vi "DDS Comms.vi"(7 "Config Folder":path, 8 "error in":errorcluster, 9 "DVR":T1, 10 "DDS Reader":refnum<class "DDS Reader.lvclass">, 11 "DDS Writer":refnum<class "DDS Writer.lvclass">) -> (0 "error out":errorcluster)   [LabVIEW 2018]
uses:
  Controls/Data Type DVRs.ctl
  <vilib>/ORNL/CSEISMIC DDS/DDS Writer/DDS Writer.lvclass
  C:/Program Files (x86)/National Instruments/LabVIEW 2018/vi.lib/ORNL/CSEISMIC DDS/CSEISMIC DDS Base/CSEISMIC DDS.lvclass
  <vilib>/ORNL/CSEISMIC DDS/DDS Reader/DDS Reader.lvclass
  <vilib>/ORNL/CSEISMIC DDS/CSEISMIC DDS Base/Data Types/IED_Status.ctl
  <vilib>/ORNL/CSEISMIC DDS/CSEISMIC DDS Base/Data Types/Controls/DeviceID.ctl
  <vilib>/ORNL/CSEISMIC DDS/CSEISMIC DDS Base/Data Types/Controls/Timestamp.ctl
  <vilib>/ORNL/CSEISMIC DDS/CSEISMIC DDS Base/Data Types/DER_Status.ctl
  <vilib>/ORNL/CSEISMIC DDS/CSEISMIC DDS Base/Data Types/Controls/DroopCurve.ctl
  <vilib>/ORNL/CSEISMIC DDS/CSEISMIC DDS Base/Data Types/DER_Info.ctl
  <vilib>/ORNL/CSEISMIC DDS/CSEISMIC DDS Base/Data Types/DER_Measurement.ctl
  <vilib>/ORNL/CSEISMIC DDS/CSEISMIC DDS Base/Data Types/ES_Info.ctl
  <vilib>/ORNL/CSEISMIC DDS/CSEISMIC DDS Base/Data Types/Controls/EfficiencyCurve.ctl
  <vilib>/ORNL/CSEISMIC DDS/CSEISMIC DDS Base/Data Types/ES_Measurement.ctl
  <vilib>/ORNL/CSEISMIC DDS/CSEISMIC DDS Base/Data Types/Generator_Info.ctl
  <vilib>/ORNL/CSEISMIC DDS/CSEISMIC DDS Base/Data Types/DER_setGenerationMode.ctl
  <vilib>/ORNL/CSEISMIC DDS/CSEISMIC DDS Base/Data Types/Controls/Generation Mode.ctl
  <vilib>/ORNL/CSEISMIC DDS/CSEISMIC DDS Base/Data Types/SmartRelay_Info.ctl
  <vilib>/ORNL/CSEISMIC DDS/CSEISMIC DDS Base/Data Types/SmartRelay_Measurement.ctl
  <vilib>/ORNL/CSEISMIC DDS/CSEISMIC DDS Base/CSEISMIC DDS.lvclass/CSEISMIC DDS.ctl
  74af6b33-939e-4f48-b39b-7a03e9a3d2c4.vi
  925c311d-217e-4777-a47a-50ede28ddcd3.vi
  1b66878a-8a8f-45b3-9ec7-57a0231460af.vi
  15938f2e-ac62-4bfc-b10c-904afcaf9918.vi
  fedd38d1-ecdd-43ef-a46f-a7af2de55406.vi
  6013e8e3-4859-43dd-bd06-f29373650741.vi
  0c0dbf40-5b73-4af0-b989-68fcfa5814cd.vi
  ee962d0e-06f6-400d-86d6-c1f49f22facc.vi
  943a1034-7167-4452-8124-675b30d37505.vi
  90619f50-e501-428c-b219-0f596dcd4826.vi
  a52a024a-1226-4015-a4cd-490690dd4f10.vi
  0e523b0e-f060-4810-9406-aaa83c92bbf0.vi
  bea21f4c-5d2d-47b9-9a7d-942307ba0c0f.vi
  88d5637e-ab37-41e7-8b27-781a427d1398.vi
  068224fe-cff3-42fe-a570-2705411094f8.vi
  62cf694c-65b3-493c-badd-292e3eb2e763.vi
  20c1c1fb-87c8-4a1b-abc1-d694dbcccceb.vi
  458aed31-5bcb-498f-bb6f-82a7e59887fc.vi
  6bb0f422-3d80-46dd-aaf7-aed45feee7e6.vi
  d6538dc3-a141-461a-88df-898e5ba76e67.vi
  <vilib>/ORNL/CSEISMIC DDS/CSEISMIC DDS Base/Accessors/Read DDS Reference.vi
  <vilib>/Utility/config.llb/Read Key (String).vi
  Global Variables/Stop (Global).vi
  <vilib>/ORNL/CSEISMIC DDS/CSEISMIC DDS Base/Error Handler.vi
  <vilib>/ORNL/CSEISMIC DDS/CSEISMIC DDS Base/CSEISMIC DDS.lvclass
  <vilib>/Utility/config.llb/NI_LVConfig.lvlib
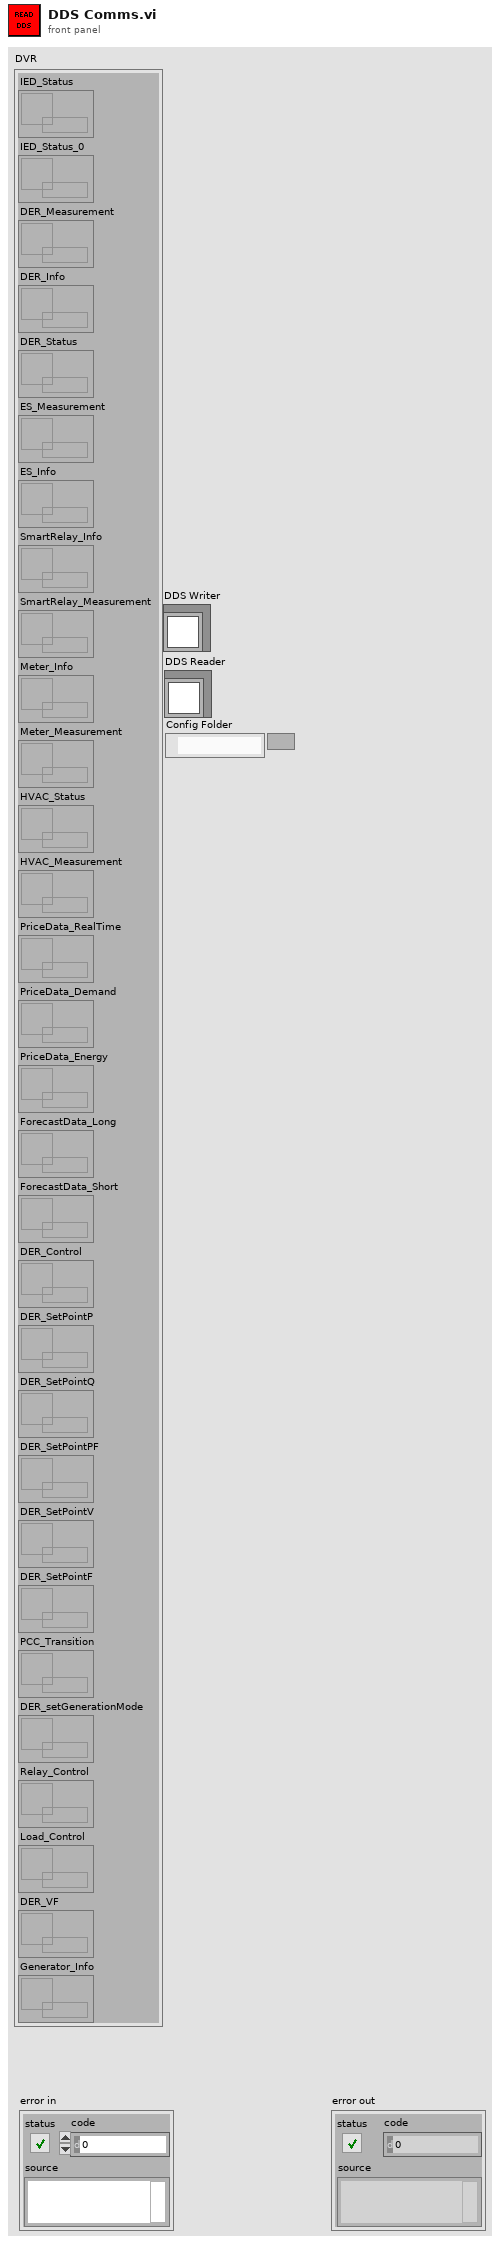
[diagram p1: front panel]
types:
  T1 = typedef "Data Type DVRs.ctl" = cluster{"IED_Status":refnum<data-value>, "IED_Status_0":refnum<data-value>, "DER_Measurement":refnum<data-value>, "DER_Info":refnum<data-value>, "DER_Status":refnum<data-value>, "ES_Measurement":refnum<data-value>, "ES_Info":refnum<data-value>, "SmartRelay_Info":refnum<data-value>, "SmartRelay_Measurement":refnum<data-value>, "Meter_Info":refnum<data-value>, "Meter_Measurement":refnum<data-value>, "HVAC_Status":refnum<data-value>, "HVAC_Measurement":refnum<data-value>, "PriceData_RealTime":refnum<data-value>, "PriceData_Demand":refnum<data-value>, "PriceData_Energy":refnum<data-value>, "ForecastData_Long":refnum<data-value>, "ForecastData_Short":refnum<data-value>, "DER_Control":refnum<data-value>, "DER_SetPointP":refnum<data-value>, "DER_SetPointQ":refnum<data-value>, "DER_SetPointPF":refnum<data-value>, "DER_SetPointV":refnum<data-value>, "DER_SetPointF":refnum<data-value>, "PCC_Transition":refnum<data-value>, "DER_setGenerationMode":refnum<data-value>, "Relay_Control":refnum<data-value>, "Load_Control":refnum<data-value>, "DER_VF":refnum<data-value>, "Generator_Info":refnum<data-value>}
  T2 = typedef "NI_LVConfig.lvlib/Config Data RefNum.ctl" = refnum<k1>
  T3 = typedef "CSEISMIC DDS.lvlib/CSEISMIC DDS.lvclass/SmartRelay_Measurement.ctl" = cluster{"DeviceID":T4, "PrimaryVoltage":dbl[], "SecondaryVoltage":dbl[], "Current":dbl[], "RealPower":dbl[], "ReactivePower":dbl[], "LineConfig":u8[], "Frequency":dbl}
  T4 = typedef "CSEISMIC DDS.lvlib/CSEISMIC DDS.lvclass/DeviceID.ctl" = string
  T5 = typedef "CSEISMIC DDS.lvlib/CSEISMIC DDS.lvclass/SmartRelay_Info.ctl" = cluster{"DeviceID":T4, "LineConfig":u8[], "NominalVoltage(V)":dbl}
  T6 = typedef "CSEISMIC DDS.lvlib/CSEISMIC DDS.lvclass/DER_setGenerationMode.ctl" = cluster{"DeviceID":T4, "Mode":T7}
  T7 = typedef "CSEISMIC DDS.lvlib/CSEISMIC DDS.lvclass/Generation Mode.ctl" = enum32{"Invalid", "PQ", "Droop", "PV", "PF", "VF"}
  T8 = typedef "CSEISMIC DDS.lvlib/CSEISMIC DDS.lvclass/Generator_Info.ctl" = cluster{"DeviceID":T4, "Voltage (V)":dbl, "MinimumPower (kVA)":dbl, "EnergyRating (kWh)":dbl, "RampRate (kW/s)":dbl, "MaxPowerFactorLeading":dbl, "MaxPowerFactorLagging":dbl, "EfficiencyCurve":T9, "StartCost":dbl, "FuelCost":dbl, "StartTime (s)":dbl}
  T9 = typedef "CSEISMIC DDS.lvlib/CSEISMIC DDS.lvclass/EfficiencyCurve.ctl" = cluster{"Power (kW)":dbl[], "Efficiency (%)":dbl[]}
  T10 = typedef "CSEISMIC DDS.lvlib/CSEISMIC DDS.lvclass/ES_Measurement.ctl" = cluster{"DeviceID":T4, "SOC (%)":dbl}
  T11 = typedef "CSEISMIC DDS.lvlib/CSEISMIC DDS.lvclass/ES_Info.ctl" = cluster{"DeviceID":T4, "EnergyRating (kWh)":dbl, "RampRate (kW/s)":dbl, "MaxPowerFactorLeading":dbl, "MaxPowerFactorLagging":dbl, "ChargingEfficiencyCurve":T9, "DischargingEfficiencyCurve":T9, "MinSOC (%)":dbl, "MaxSOC (%)":dbl}
  T12 = typedef "CSEISMIC DDS.lvlib/CSEISMIC DDS.lvclass/DER_Measurement.ctl" = cluster{"DeviceID":T4, "Voltage":dbl[], "Current":dbl[], "RealPower":dbl[], "ReactivePower":dbl[], "LineConfig":u8[], "Frequency":dbl}
  T13 = typedef "CSEISMIC DDS.lvlib/CSEISMIC DDS.lvclass/DER_Info.ctl" = cluster{"DeviceID":T4, "LineConfig":u8[], "NominalVoltage(V)":dbl, "PowerRating(kVA)":dbl, "VFControl":bool, "PControl":bool, "QControl":bool, "PFControl":bool, "PVControl":bool, "Droop":bool, "DroopConfigurable":bool, "Unbalanced":bool}
  T14 = typedef "CSEISMIC DDS.lvlib/CSEISMIC DDS.lvclass/DER_Status.ctl" = cluster{"DeviceID":T4, "VFControl":bool, "PControl":bool, "QControl":bool, "PFControl":bool, "PVControl":bool, "Droop":bool, "Unbalanced":bool, "MicrogridVF":bool, "RealDroop(kW)":T15, "ReactiveDroop(kVar)":T15}
  T15 = typedef "CSEISMIC DDS.lvlib/CSEISMIC DDS.lvclass/DroopCurve.ctl" = cluster{"XMin":dbl, "XMax":dbl, "YMin":dbl, "YMax":dbl}
  T16 = typedef "CSEISMIC DDS.lvlib/CSEISMIC DDS.lvclass/IED_Status.ctl" = cluster{"DeviceID":T4, "Timestamp":T17, "MicrogridID":u8, "Active":bool, "Inactive":bool, "Error":i32, "Fault":bool, "ErrorString":string}
  T17 = typedef "CSEISMIC DDS.lvlib/CSEISMIC DDS.lvclass/Timestamp.ctl" = cluster{"Seconds":u64, "Remainder":u64}
  T18 = typedef "CSEISMIC DDS.lvlib/CSEISMIC DDS.lvclass/DER_Control.ctl" = cluster{"DeviceID":T4, "Activate":bool, "Deactivate":bool}
  T19 = typedef "LVDDS_library.lvlib/DDS Sample Info.ctl" = cluster{"DDS_SampleStateKind":enum32{"DDS_INVALID_SAMPLE_STATE", "DDS_READ_SAMPLE_STATE", "DDS_NOT_READ_SAMPLE_STATE"}, "DDS_ViewStateKind":enum32{"DDS_INVALID_SAMPLE_STATE", "DDS_NEW_VIEW_STATE", "DDS_NOT_NEW_VIEW_STATE"}, "DDS_InstanceStateKind":enum32{"DDS_INVALID_STATE", "DDS_ALIVE_INSTANCE_STATE", "DDS_NOT_ALIVE_DISPOSED_INSTANCE_STATE", "", "DDS_NOT_ALIVE_NO_WRITERS_INSTANCE_STATE"}, "sec":i32, "nanosec":u32, "valid_data":bool}
  T20 = typedef "CSEISMIC DDS.lvlib/CSEISMIC DDS.lvclass/PCC_Transition.ctl" = cluster{"DeviceID":T4, "Island":bool, "Resynchronize":bool}
  T21 = typedef "CSEISMIC DDS.lvlib/CSEISMIC DDS.lvclass/DER_SetPointP.ctl" = cluster{"DeviceID":T4, "RealPower (kW)":dbl[]}
  T22 = typedef "CSEISMIC DDS.lvlib/CSEISMIC DDS.lvclass/DER_SetPointQ.ctl" = cluster{"DeviceID":T4, "ReactivePower (kVAR)":dbl[]}
  T23 = typedef "CSEISMIC DDS.lvlib/CSEISMIC DDS.lvclass/DER_SetPointF.ctl" = cluster{"DeviceID":T4, "Frequency (Hz)":dbl}
  T24 = typedef "CSEISMIC DDS.lvlib/CSEISMIC DDS.lvclass/DER_SetPointV.ctl" = cluster{"DeviceID":T4, "Voltage (V)":dbl}
  T25 = typedef "CSEISMIC DDS.lvlib/CSEISMIC DDS.lvclass/DER_VF.ctl" = cluster{"DeviceID":T4}
  T26 = typedef "CSEISMIC DDS.lvlib/CSEISMIC DDS.lvclass/Relay_Control.ctl" = cluster{"DeviceID":T4, "Activate":bool, "Deactivate":bool}
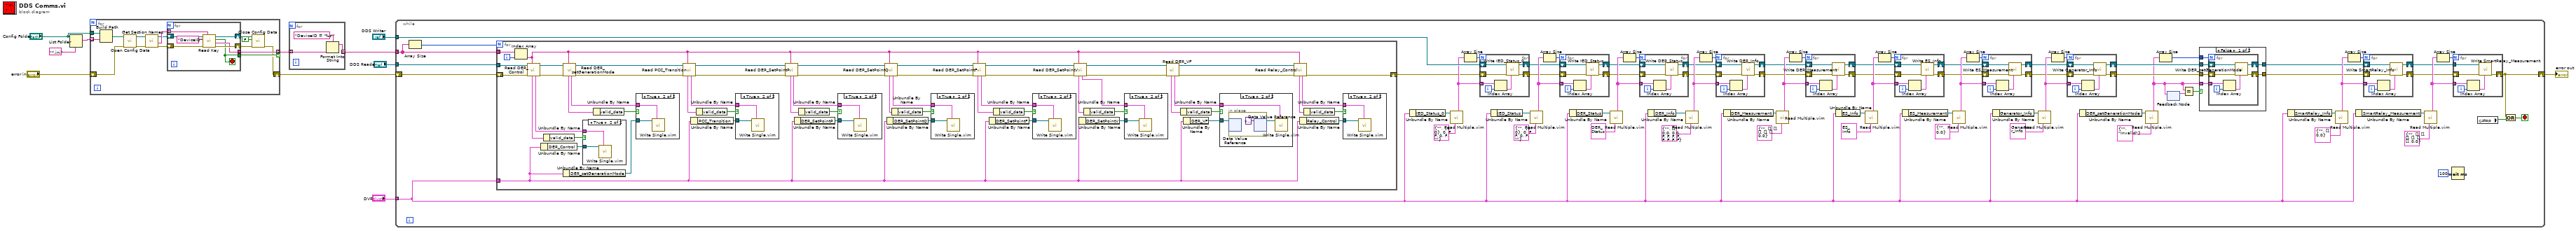
[diagram p0: block diagram]
diagram:
  n1 = List Folder(path="Config Folder", pattern="*.ini") -> (filenames=w5:string[])  [unwired: 2 in, 3 out]
  n2 = for {
    tunnel: w5 -> [w25] mode=indexing
    tunnel: "Config Folder" -> [w26]
    shift-right: [w13] -> w1
    shift-left: "error in" -> [w21]
    tunnel: [w17] -> w2 mode=indexing if=w14
    n3 = Build Path(base path=w26, name or relative path=w25) -> (appended path=w22:path)
    n4 = call <vilib>:"Open Config Data.vi"("error in (no error)"=w21, "configuration file path"=w22) -> ("error out"=w24:errorcluster, "refnum"=w23:T2)  [unwired: 7 in, 1 out]
    n5 = call <vilib>:"Get Section Names.vi"("error in (no error)"=w24, "refnum"=w23) -> ("error out"=w18:errorcluster, "section names"=w20:string[], "refnum out"=w19:T2)  [unwired: 7 in]
    n6 = for {
      tunnel: w20 -> [w34] mode=indexing
      shift-right: [w30] -> w16
      shift-left: w19 -> [w33]
      shift-right: [w31] -> w15
      shift-left: w18 -> [w32]
      tunnel: [w28] -> w17
      tunnel: [w27] -> w14
      stop <- w27 stop-if-true
      n7 = call-poly <vilib>:"Read Key.vi"("section"=w34, "error in (no error)"=w32, "key"="DeviceID", "refnum"=w33) -> ("error out"=w31:errorcluster, "value"=w28:string, "found?"=w27:bool, "refnum out"=w30:T2)  [unwired: 4 in]
    }
    n8 = call <vilib>:"Close Config Data.vi"("error in (no error)"=w15, "write file if changed (T)"=FALSE, "refnum"=w16) -> ("error out"=w13:errorcluster)  [unwired: 7 in, 1 out]
  }
  n9 = for {
    tunnel: w2 -> [w36] mode=indexing
    tunnel: [w35] -> w7 mode=indexing
    n10 = Format Into String(format string="DeviceID = '%s'" ("Query condition"), w36) -> (resulting string=w35:string)  [unwired: 2 in, 1 out]
  }
  n11 = while {
    tunnel: "DDS Reader" -> [w114]
    tunnel: "DDS Writer" -> [w112]
    tunnel: "DVR" -> [w93]
    shift-right: [w41] -> w10
    shift-left: w1 -> [w113]
    tunnel: w7 -> [w85]
    stop <- w87 stop-if-true
    n12 = Array Size(array=w85) -> (size(s)=w84:i32)
    n13 = for {
      N: w84 -> [_]
      tunnel: w114 -> [w171]
      tunnel: w93 -> [w116]
      shift-right: [w129] -> w70
      shift-left: w113 -> [w128]
      tunnel: w85 -> [w127]
      i -> [w126]
      n14 = Index Array(array=w127, index=w126) -> (element=w119:string)
      n15 = call <vilib>:"Read DER_Control.vi"("Query condition"=w119, "error in"=w128, "DDS Reader in"=w171) -> ("error out"=w173:errorcluster, "DDS Reader out"=w172:refnum<class "DDS Reader.lvclass">, "data"=w157:T18, "DDS Sample Info"=w159:T19)  [unwired: 5 in]
      n16 = Unbundle By Name(w116) -> ("DER_Control"=w160:refnum<data-value>)
      n17 = Unbundle By Name(w159) -> ("valid_data"=w158:bool)
      n18 = Unbundle By Name(w116) -> ("DER_setGenerationMode"=w155:refnum<data-value>)
      n19 = call <vilib>:"Read DER_setGenerationMode.vi"("Query condition"=w119, "error in"=w173, "DDS Reader in"=w172) -> ("error out"=w169:errorcluster, "DDS Reader out"=w170:refnum<class "DDS Reader.lvclass">, "data"=w154:T6, "DDS Sample Info"=w153:T19)  [unwired: 5 in]
      n20 = case shown="True" w158 {
        tunnel: w160 -> [_ w191]
        tunnel: w157 -> [_ w190]
        frame False {
        }
        frame True {
          n21 = call "Write Single.vim"("Data Element"=w190, "Data DVR"=w191) -> ()  [unwired: 9 in, 1 out]
        }
      }
      n22 = Unbundle By Name(w153) -> ("valid_data"=w156:bool)
      n23 = case shown="True" w156 {
        tunnel: w155 -> [_ w189]
        tunnel: w154 -> [_ w188]
        frame False {
        }
        frame True {
          n24 = call "Write Single.vim"("Data Element"=w188, "Data DVR"=w189) -> ()  [unwired: 9 in, 1 out]
        }
      }
      n25 = call <vilib>:"Read PCC_Transition.vi"("Query condition"=w119, "error in"=w169, "DDS Reader in"=w170) -> ("error out"=w168:errorcluster, "DDS Reader out"=w167:refnum<class "DDS Reader.lvclass">, "data"=w150:T20, "DDS Sample Info"=w149:T19)  [unwired: 5 in]
      n26 = Unbundle By Name(w116) -> ("PCC_Transition"=w151:refnum<data-value>)
      n27 = Unbundle By Name(w149) -> ("valid_data"=w152:bool)
      n28 = case shown="True" w152 {
        tunnel: w151 -> [_ w183]
        tunnel: w150 -> [_ w182]
        frame False {
        }
        frame True {
          n29 = call "Write Single.vim"("Data Element"=w182, "Data DVR"=w183) -> ()  [unwired: 9 in, 1 out]
        }
      }
      n30 = call <vilib>:"Read DER_SetPointP.vi"("Query condition"=w119, "error in"=w168, "DDS Reader in"=w167) -> ("error out"=w165:errorcluster, "DDS Reader out"=w166:refnum<class "DDS Reader.lvclass">, "data"=w146:T21, "DDS Sample Info"=w145:T19)  [unwired: 5 in]
      n31 = Unbundle By Name(w116) -> ("DER_SetPointP"=w148:refnum<data-value>)
      n32 = Unbundle By Name(w145) -> ("valid_data"=w147:bool)
      n33 = case shown="True" w147 {
        tunnel: w148 -> [_ w181]
        tunnel: w146 -> [_ w180]
        frame False {
        }
        frame True {
          n34 = call "Write Single.vim"("Data Element"=w180, "Data DVR"=w181) -> ()  [unwired: 9 in, 1 out]
        }
      }
      n35 = call <vilib>:"Read DER_SetPointQ.vi"("Query condition"=w119, "error in"=w165, "DDS Reader in"=w166) -> ("error out"=w163:errorcluster, "DDS Reader out"=w164:refnum<class "DDS Reader.lvclass">, "data"=w142:T22, "DDS Sample Info"=w141:T19)  [unwired: 5 in]
      n36 = Unbundle By Name(w116) -> ("DER_SetPointQ"=w143:refnum<data-value>)
      n37 = Unbundle By Name(w141) -> ("valid_data"=w144:bool)
      n38 = case shown="True" w144 {
        tunnel: w143 -> [_ w185]
        tunnel: w142 -> [_ w184]
        frame False {
        }
        frame True {
          n39 = call "Write Single.vim"("Data Element"=w184, "Data DVR"=w185) -> ()  [unwired: 9 in, 1 out]
        }
      }
      n40 = call <vilib>:"Read DER_SetPointF.vi"("Query condition"=w119, "error in"=w163, "DDS Reader in"=w164) -> ("error out"=w121:errorcluster, "DDS Reader out"=w123:refnum<class "DDS Reader.lvclass">, "data"=w115:T23, "DDS Sample Info"=w138:T19)  [unwired: 5 in]
      n41 = Unbundle By Name(w116) -> ("DER_SetPointF"=w140:refnum<data-value>)
      n42 = Unbundle By Name(w138) -> ("valid_data"=w139:bool)
      n43 = case shown="True" w139 {
        tunnel: w140 -> [_ w187]
        tunnel: w115 -> [_ w186]
        frame False {
        }
        frame True {
          n44 = call "Write Single.vim"("Data Element"=w186, "Data DVR"=w187) -> ()  [unwired: 9 in, 1 out]
        }
      }
      n45 = call <vilib>:"Read DER_SetPointV.vi"("Query condition"=w119, "error in"=w121, "DDS Reader in"=w123) -> ("error out"=w120:errorcluster, "DDS Reader out"=w122:refnum<class "DDS Reader.lvclass">, "data"=w117:T24, "DDS Sample Info"=w118:T19)  [unwired: 5 in]
      n46 = Unbundle By Name(w116) -> ("DER_SetPointV"=w124:refnum<data-value>)
      n47 = Unbundle By Name(w118) -> ("valid_data"=w125:bool)
      n48 = case shown="True" w125 {
        tunnel: w124 -> [_ w175]
        tunnel: w117 -> [_ w174]
        frame False {
        }
        frame True {
          n49 = call "Write Single.vim"("Data Element"=w174, "Data DVR"=w175) -> ()  [unwired: 9 in, 1 out]
        }
      }
      n50 = call <vilib>:"Read DER_VF.vi"("error in"=w120, "DDS Reader in"=w122) -> ("error out"=w161:errorcluster, "DDS Reader out"=w162:refnum<class "DDS Reader.lvclass">, "data"=w135:T25, "DDS Sample Info"=w134:T19)  [unwired: 6 in]
      n51 = Unbundle By Name(w134) -> ("valid_data"=w137:bool)
      n52 = Unbundle By Name(w116) -> ("DER_VF"=w136:refnum<data-value>)
      n53 = case shown="True" w137 {
        tunnel: w136 -> [_ w177]
        tunnel: w135 -> [_ w178]
        frame False {
        }
        frame True {
          n54 = in-place {
            n55 = in-place-dvr #1(w177) -> ()  [unwired: 2 out]
            n56 = in-place-dvr #1(variant ("data value")) -> (w176:refnum<data-value>)  [unwired: 1 out]
          }
          n57 = call "Write Single.vim"("Data Element"=w178, "Data DVR"=w176) -> ()  [unwired: 9 in, 1 out]
        }
      }
      n58 = call <vilib>:"Read Relay_Control.vi"("Query condition"=w119, "error in"=w161, "DDS Reader in"=w162) -> ("error out"=w129:errorcluster, "data"=w131:T26, "DDS Sample Info"=w130:T19)  [unwired: 5 in, 1 out]
      n59 = Unbundle By Name(w116) -> ("Relay_Control"=w133:refnum<data-value>)
      n60 = Unbundle By Name(w130) -> ("valid_data"=w132:bool)
      n61 = case shown="True" w132 {
        tunnel: w133 -> [_ w193]
        tunnel: w131 -> [_ w192]
        frame False {
        }
        frame True {
          n62 = call "Write Single.vim"("Data Element"=w192, "Data DVR"=w193) -> ()  [unwired: 9 in, 1 out]
        }
      }
    }
    n63 = Unbundle By Name(w93) -> ("IED_Status_0"=w110:refnum<data-value>)
    n64 = call "Read Multiple.vim"("Data Type"=T16 {"DeviceID"="", "Timestamp"={"Seconds"=0, "Remainder"=0}, "MicrogridID"=0, "Active"=FALSE, "Inactive"=FALSE, "Error"=0, "Fault"=FALSE, "ErrorString"=""} ("IED_Status"), "Data DVR"=w110) -> ("Data Array"=w83:T16[])  [unwired: 8 in, 1 out]
    n65 = Array Size(array=w83) -> (size(s)=w82:i32)
    n66 = for {
      N: w82 -> [_]
      shift-right: [w271] -> w69
      shift-left: w70 -> [w269]
      shift-right: [w270] -> w68
      shift-left: w112 -> [w268]
      tunnel: w83 -> [w267]
      i -> [w266]
      n67 = Index Array(array=w267, index=w266) -> (element=w265:T16)
      n68 = call <vilib>:"Write IED_Status_0.vi"("IED_Status"=w265, "error in"=w269, "DDS Writer in"=w268) -> ("error out"=w271:errorcluster, "DDS Writer out"=w270:refnum<class "DDS Writer.lvclass">)  [unwired: 7 in]
    }
    n69 = Unbundle By Name(w93) -> ("IED_Status"=w109:refnum<data-value>)
    n70 = call "Read Multiple.vim"("Data Type"=T16 {"DeviceID"="", "Timestamp"={"Seconds"=0, "Remainder"=0}, "MicrogridID"=0, "Active"=FALSE, "Inactive"=FALSE, "Error"=0, "Fault"=FALSE, "ErrorString"=""} ("IED_Status"), "Data DVR"=w109) -> ("Data Array"=w71:T16[])  [unwired: 8 in, 1 out]
    n71 = Array Size(array=w71) -> (size(s)=w81:i32)
    n72 = for {
      N: w81 -> [_]
      shift-right: [w264] -> w58
      shift-left: w69 -> [w262]
      shift-right: [w263] -> w59
      shift-left: w68 -> [w261]
      tunnel: w71 -> [w260]
      i -> [w259]
      n73 = Index Array(array=w260, index=w259) -> (element=w258:T16)
      n74 = call <vilib>:"Write IED_Status.vi"("IED_Status"=w258, "error in"=w262, "DDS Writer in"=w261) -> ("error out"=w264:errorcluster, "DDS Writer out"=w263:refnum<class "DDS Writer.lvclass">)  [unwired: 7 in]
    }
    n75 = Unbundle By Name(w93) -> ("DER_Status"=w107:refnum<data-value>)
    n76 = call "Read Multiple.vim"("Data Type"=T14 {"DeviceID"="", "VFControl"=FALSE, "PControl"=FALSE, "QControl"=FALSE, "PFControl"=FALSE, "PVControl"=FALSE, "Droop"=FALSE, "Unbalanced"=FALSE, "MicrogridVF"=FALSE, "RealDroop(kW)"={"XMin"=0.0, "XMax"=0.0, "YMin"=0.0, "YMax"=0.0}, "ReactiveDroop(kVar)"={"XMin"=0.0, "XMax"=0.0, "YMin"=0.0, "YMax"=0.0}} ("DER_Status"), "Data DVR"=w107) -> ("Data Array"=w67:T14[])  [unwired: 8 in, 1 out]
    n77 = Array Size(array=w67) -> (size(s)=w80:i32)
    n78 = for {
      N: w80 -> [_]
      shift-right: [w257] -> w57
      shift-left: w58 -> [w255]
      shift-right: [w256] -> w56
      shift-left: w59 -> [w254]
      tunnel: w67 -> [w253]
      i -> [w252]
      n79 = Index Array(array=w253, index=w252) -> (element=w251:T14)
      n80 = call <vilib>:"Write DER_Status.vi"("DER_Status"=w251, "error in"=w255, "DDS Writer in"=w254) -> ("error out"=w257:errorcluster, "DDS Writer out"=w256:refnum<class "DDS Writer.lvclass">)  [unwired: 7 in]
    }
    n81 = Unbundle By Name(w93) -> ("DER_Info"=w106:refnum<data-value>)
    n82 = call "Read Multiple.vim"("Data Type"=T13 {"DeviceID"="", "LineConfig"=[], "NominalVoltage(V)"=0.0, "PowerRating(kVA)"=0.0, "VFControl"=FALSE, "PControl"=FALSE, "QControl"=FALSE, "PFControl"=FALSE, "PVControl"=FALSE, "Droop"=FALSE, "DroopConfigurable"=FALSE, "Unbalanced"=FALSE} ("DER_Info"), "Data DVR"=w106) -> ("Data Array"=w66:T13[])  [unwired: 8 in, 1 out]
    n83 = Array Size(array=w66) -> (size(s)=w79:i32)
    n84 = for {
      N: w79 -> [_]
      shift-right: [w250] -> w54
      shift-left: w57 -> [w248]
      shift-right: [w249] -> w55
      shift-left: w56 -> [w247]
      tunnel: w66 -> [w246]
      i -> [w245]
      n85 = Index Array(array=w246, index=w245) -> (element=w244:T13)
      n86 = call <vilib>:"Write DER_Info.vi"("DER_Info"=w244, "error in"=w248, "DDS Writer in"=w247) -> ("error out"=w250:errorcluster, "DDS Writer out"=w249:refnum<class "DDS Writer.lvclass">)  [unwired: 7 in]
    }
    n87 = Unbundle By Name(w93) -> ("DER_Measurement"=w105:refnum<data-value>)
    n88 = call "Read Multiple.vim"("Data Type"=T12 {"DeviceID"="", "Voltage"=[], "Current"=[], "RealPower"=[], "ReactivePower"=[], "LineConfig"=[], "Frequency"=0.0} ("DER_Measurement"), "Data DVR"=w105) -> ("Data Array"=w65:T12[])  [unwired: 8 in, 1 out]
    n89 = Array Size(array=w65) -> (size(s)=w78:i32)
    n90 = for {
      N: w78 -> [_]
      shift-right: [w243] -> w53
      shift-left: w54 -> [w241]
      shift-right: [w242] -> w52
      shift-left: w55 -> [w240]
      tunnel: w65 -> [w239]
      i -> [w238]
      n91 = Index Array(array=w239, index=w238) -> (element=w237:T12)
      n92 = call <vilib>:"Write DER_Measurement.vi"("DER_Measurement"=w237, "error in"=w241, "DDS Writer in"=w240) -> ("error out"=w243:errorcluster, "DDS Writer out"=w242:refnum<class "DDS Writer.lvclass">)  [unwired: 7 in]
    }
    n93 = Unbundle By Name(w93) -> ("ES_Info"=w103:refnum<data-value>)
    n94 = call "Read Multiple.vim"("Data Type"=T11 {"DeviceID"="", "EnergyRating (kWh)"=0.0, "RampRate (kW/s)"=0.0, "MaxPowerFactorLeading"=0.0, "MaxPowerFactorLagging"=0.0, "ChargingEfficiencyCurve"={"Power (kW)"=[], "Efficiency (%)"=[]}, "DischargingEfficiencyCurve"={"Power (kW)"=[], "Efficiency (%)"=[]}, "MinSOC (%)"=0.0, "MaxSOC (%)"=0.0} ("ES_Info"), "Data DVR"=w103) -> ("Data Array"=w64:T11[])  [unwired: 8 in, 1 out]
    n95 = Array Size(array=w64) -> (size(s)=w77:i32)
    n96 = for {
      N: w77 -> [_]
      shift-right: [w236] -> w51
      shift-left: w53 -> [w234]
      shift-right: [w235] -> w50
      shift-left: w52 -> [w233]
      tunnel: w64 -> [w232]
      i -> [w231]
      n97 = Index Array(array=w232, index=w231) -> (element=w230:T11)
      n98 = call <vilib>:"Write ES_Info.vi"("ES_Info"=w230, "error in"=w234, "DDS Writer in"=w233) -> ("error out"=w236:errorcluster, "DDS Writer out"=w235:refnum<class "DDS Writer.lvclass">)  [unwired: 7 in]
    }
    n99 = Unbundle By Name(w93) -> ("ES_Measurement"=w104:refnum<data-value>)
    n100 = call "Read Multiple.vim"("Data Type"=T10 {"DeviceID"="", "SOC (%)"=0.0} ("ES_Measurement"), "Data DVR"=w104) -> ("Data Array"=w63:T10[])  [unwired: 8 in, 1 out]
    n101 = Array Size(array=w63) -> (size(s)=w76:i32)
    n102 = for {
      N: w76 -> [_]
      shift-right: [w229] -> w48
      shift-left: w51 -> [w227]
      shift-right: [w228] -> w49
      shift-left: w50 -> [w226]
      tunnel: w63 -> [w225]
      i -> [w224]
      n103 = Index Array(array=w225, index=w224) -> (element=w223:T10)
      n104 = call <vilib>:"Write ES_Measurement.vi"("ES_Measurement"=w223, "error in"=w227, "DDS Writer in"=w226) -> ("error out"=w229:errorcluster, "DDS Writer out"=w228:refnum<class "DDS Writer.lvclass">)  [unwired: 7 in]
    }
    n105 = Unbundle By Name(w93) -> ("Generator_Info"=w97:refnum<data-value>)
    n106 = call "Read Multiple.vim"("Data Type"=T8 {"DeviceID"="", "Voltage (V)"=0.0, "MinimumPower (kVA)"=0.0, "EnergyRating (kWh)"=0.0, "RampRate (kW/s)"=0.0, "MaxPowerFactorLeading"=0.0, "MaxPowerFactorLagging"=0.0, "EfficiencyCurve"={"Power (kW)"=[], "Efficiency (%)"=[]}, "StartCost"=0.0, "FuelCost"=0.0, "StartTime (s)"=0.0} ("Generator_Info"), "Data DVR"=w97) -> ("Data Array"=w62:T8[])  [unwired: 8 in, 1 out]
    n107 = Array Size(array=w62) -> (size(s)=w75:i32)
    n108 = for {
      N: w75 -> [_]
      shift-right: [w222] -> w47
      shift-left: w48 -> [w220]
      shift-right: [w221] -> w46
      shift-left: w49 -> [w219]
      tunnel: w62 -> [w218]
      i -> [w217]
      n109 = Index Array(array=w218, index=w217) -> (element=w216:T8)
      n110 = call <vilib>:"Write Generator_Info.vi"("Generator_Info"=w216, "error in"=w220, "DDS Writer in"=w219) -> ("error out"=w222:errorcluster, "DDS Writer out"=w221:refnum<class "DDS Writer.lvclass">)  [unwired: 7 in]
    }
    n111 = Unbundle By Name(w93) -> ("DER_setGenerationMode"=w96:refnum<data-value>)
    n112 = call "Read Multiple.vim"("Data Type"=T6 {"DeviceID"="", "Mode"=enum."Invalid"} ("DER_setGenerationMode"), "Data DVR"=w96) -> ("Data Array"=w38:T6[])  [unwired: 8 in, 1 out]
    n113 = Array Size(array=w38) -> (size(s)=w74:i32)
    n114 = feedback #2() -> (w40:T6[])  [unwired: 1 in]
    n115 = feedback-in #2(w38) -> ()
    n116 = Equal?(x=w38, y=w40) -> (x = y?=w39:bool)
    n117 = case shown="False" w39 {
      tunnel: w74 -> [w199 _]
      tunnel: w38 -> [w198 _]
      tunnel: w47 -> [w197 w207]
      tunnel: w46 -> [w196 w208]
      tunnel: [w195 w208] -> w45
      tunnel: [w194 w207] -> w44
      frame False {
        n118 = for {
          N: w199 -> [_]
          shift-right: [w206] -> w194
          shift-left: w197 -> [w204]
          shift-right: [w205] -> w195
          shift-left: w196 -> [w203]
          tunnel: w198 -> [w202]
          i -> [w201]
          n119 = Index Array(array=w202, index=w201) -> (element=w200:T6)
          n120 = call <vilib>:"Write DER_setGenerationMode.vi"("DER_setGenerationMode"=w200, "error in"=w204, "DDS Writer in"=w203) -> ("error out"=w206:errorcluster, "DDS Writer out"=w205:refnum<class "DDS Writer.lvclass">)  [unwired: 7 in]
        }
      }
      frame True {
      }
    }
    n121 = Unbundle By Name(w93) -> ("SmartRelay_Info"=w94:refnum<data-value>)
    n122 = call "Read Multiple.vim"("Data Type"=T5 {"DeviceID"="", "LineConfig"=[], "NominalVoltage(V)"=0.0} ("SmartRelay_Info"), "Data DVR"=w94) -> ("Data Array"=w61:T5[])  [unwired: 8 in, 1 out]
    n123 = Array Size(array=w61) -> (size(s)=w73:i32)
    n124 = Unbundle By Name(w93) -> ("SmartRelay_Measurement"=w95:refnum<data-value>)
    n125 = for {
      N: w73 -> [_]
      shift-right: [w215] -> w42
      shift-left: w44 -> [w213]
      shift-right: [w214] -> w43
      shift-left: w45 -> [w212]
      tunnel: w61 -> [w211]
      i -> [w210]
      n126 = Index Array(array=w211, index=w210) -> (element=w209:T5)
      n127 = call <vilib>:"Write SmartRelay_Info.vi"("SmartRelay_Info"=w209, "error in"=w213, "DDS Writer in"=w212) -> ("error out"=w215:errorcluster, "DDS Writer out"=w214:refnum<class "DDS Writer.lvclass">)  [unwired: 7 in]
    }
    n128 = call "Read Multiple.vim"("Data Type"=T3 {"DeviceID"="", "PrimaryVoltage"=[], "SecondaryVoltage"=[], "Current"=[], "RealPower"=[], "ReactivePower"=[], "LineConfig"=[], "Frequency"=0.0} ("SmartRelay_Measurement"), "Data DVR"=w95) -> ("Data Array"=w60:T3[])  [unwired: 8 in, 1 out]
    n129 = Array Size(array=w60) -> (size(s)=w72:i32)
    n130 = Wait (ms)(milliseconds to wait=u32 100) -> ()  [unwired: 1 out]
    n131 = for {
      N: w72 -> [_]
      shift-right: [w277] -> w41
      shift-left: w42 -> [w276]
      tunnel: w60 -> [w274]
      tunnel: w43 -> [w275]
      i -> [w273]
      n132 = Index Array(array=w274, index=w273) -> (element=w272:T3)
      n133 = call <vilib>:"Write SmartRelay_Measurement.vi"("SmartRelay_Measurement"=w272, "error in"=w276, "DDS Writer in"=w275) -> ("error out"=w277:errorcluster)  [unwired: 7 in, 1 out]
    }
    n134 = global read "Stop (Global).vi" "stop"() -> (w88:bool)
    n135 = Or(x=w41, y=w88) -> (x .or. y?=w87:bool)
  }
  "error out" <- w10
